vi "Add Entity.vi"(8 "error in (no error)":errorcluster, 9 "Table Name":string, 10 "Entity":refnum<class "Entity.lvclass">, 11 "EntityPersistMap in":refnum<class "EntityPersistMap.lvclass">) -> (0 "error out":errorcluster, 2 "New?":bool, 3 "EntityPersistMap out":refnum<class "EntityPersistMap.lvclass">)   [LabVIEW 2020, in "Conditum SQLite.lvlib" / "EntityPersistMap.lvclass"]
uses:
  EntityPersistMap.lvclass
  EntityPersistMap.lvclass/EntityPersistMap.ctl
  <vilib>/IlluminatedG/IG Conditum Base/Conditum/Entity/Entity.lvclass
  <vilib>/Utility/miscctls.llb/LVMapReplaceAction.ctl
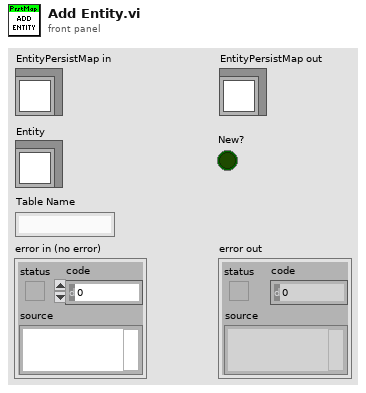
[diagram p1: front panel]
types:
  T1 = typedef "LVMapReplaceAction.ctl" = enum32{"Modify Entry only if found", "Add or Modify Entry", "Delete Entry"}
  T2 = typedef "Conditum.lvlib/Entity ID.ctl" = i64
  T3 = map{string, map{T2, refnum<class "Entity.lvclass">}}
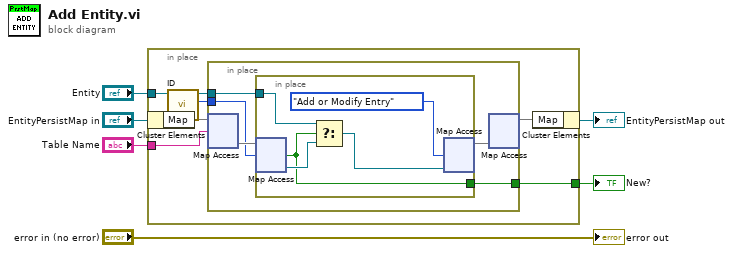
[diagram p0: block diagram]
diagram:
  n1 = in-place {
    in-place-border: "Table Name" -> [w12]
    in-place-border: "Entity" -> [w11]
    in-place-border: [w8] -> w2
    n2 = in-place-cluster #1("EntityPersistMap in") -> ("Map"=w13:T3)
    n3 = call <vilib>:"ID.vi"("Entity in"=w11) -> ("ID"=w9:T2, "Entity out"=w10:refnum<class "Entity.lvclass">)  [unwired: 9 in]
    n4 = in-place {
      in-place-border: w10 -> [w18]
      in-place-border: w9 -> [w16]
      in-place-border: [w15] -> w8
      n5 = in-place-map #2(w13, w12) -> (w17:map{T2, refnum<class "Entity.lvclass">})  [unwired: 1 in, 1 out]
      n6 = in-place {
        in-place-border: w18 -> [w21]
        in-place-border: [w22] -> w15
        n7 = in-place-map #3(w17, w16) -> (w23:refnum<class "Entity.lvclass">, w22:bool)  [unwired: 1 in]
        n8 = Select(t=w21, s=w22, f=w23) -> (s? t:f=w20:refnum<class "Entity.lvclass">)
        n9 = in-place-map #3(w20, LVMapReplaceAction."Add or Modify Entry" ("action")) -> (w14:map{T2, refnum<class "Entity.lvclass">})  [unwired: 2 out]
      }
      n10 = in-place-map #2(w14) -> (w7:T3)  [unwired: 1 in, 2 out]
    }
    n11 = in-place-cluster #1("Map"=w7) -> (→"EntityPersistMap out":refnum<class "EntityPersistMap.lvclass">)
  }
  "New?" <- w2
  "error out" <- "error in (no error)"
